vi "LEP_RV_WordWrap.vi"(10 "width":u32=270, 11 "input string":string="1 2 3 4 5 6 7 8 9 1 2 3 4 5 6 7 8 1 2 3 4 5 6 7 8 9 1 2 3 4 5 6 7 8 1 2 3 4 5 6 7 8 9 1 2 3 4 5 6 7 8 1 2 3 4 5 6 7 8 9 1 2 3 4 5 6 7 8 1 2 3 4 5 6 7 8 9 1 2 3 4 5 6 7 8 1 2 3 4 5 6 7 8 9 1 2 3 4 5 6 7 8 1 2 3 4 5 6 7 8 9 1 2 3 4 5 6 7 8 1 2 3 4 5 6 7 8 9 1 2 3 4 5 6 7 8") -> (3 "output string":string)   [LabVIEW 2011]
panel:
  out "width control":string
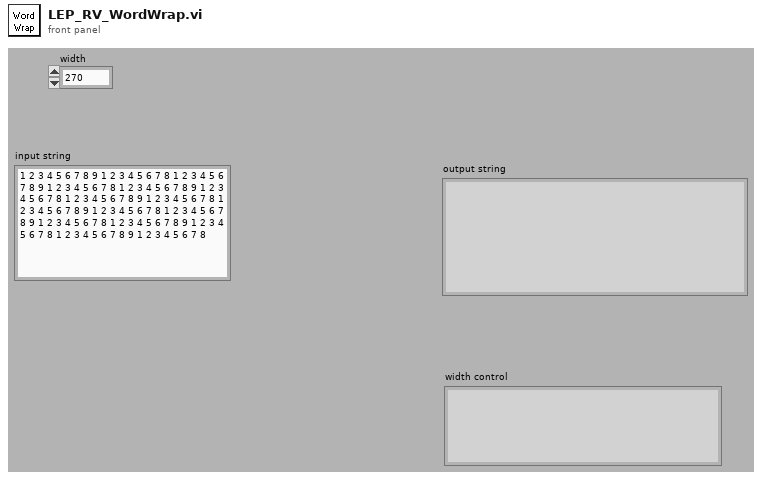
[diagram p1: front panel]
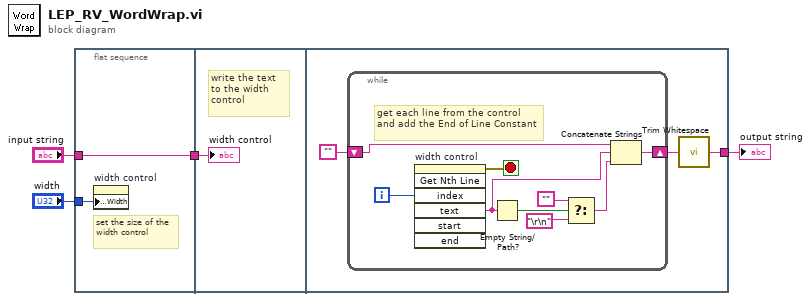
[diagram p0: block diagram]
diagram:
  n1 = flat-sequence {
    tunnel: "width" -> [w6]
    tunnel: "input string" -> [w5]
    tunnel: [w5] -> w4
    tunnel: w4 -> [w7]
    tunnel: [w8] -> w1
    frame #0 {
      # "set the size of the width control"
      n2 = property on="width control" class="Str"("Text Size:Width"=w6) -> ()  [unwired: 2 in, 2 out]
    }
    frame #1 {
      # "write the text to the width control"
      "width control" <- w7
    }
    frame #2 {
      n3 = while {
        shift-right: [w12] -> w9
        shift-left: "" ("Empty String Constant") -> [w18]
        i -> [w11]
        stop <- w19 stop-if-true
        # "get each line from the control and add the End of Line Constant"
        n4 = invoke on="width control" class="Str" method="Get Nth Line"("index"=w11) -> (error out=w19:errorcluster, "text"=w14:string)  [unwired: 6 in, 5 out]
        n5 = Empty String/Path?(string/path=w14) -> (empty?=w15:bool)
        n6 = Select(t="" ("Empty String Constant"), s=w15, f="\r\n" ("End of Line Constant")) -> (s? t:f=w13:string)
        n7 = Concatenate Strings(w18, w14, w13) -> (w12:string)
      }
      n8 = call <vilib>:"Trim Whitespace.vi"("string"=w9) -> ("trimmed string"=w8:string)  [unwired: 1 in]
    }
  }
  "output string" <- w1
